vi "_DeviceCommandsInfo.vi"(0 "device name":string) -> (1 "error_stack":string[](array[string]), 2 "commands_info":T1(array[cluster]), 3 "success":bool=TRUE)   [LabVIEW 2014, in "tango.lvlib"]
uses:
  tango.lvlib
  tango_binding.so
panel:
  out "error_stack":string[](array[string])
  out "success":bool
  # "CommandInfo.level\n-----------------------\n\tOPERATOR = 0\n EXPERT = 1"
  # "CommandInfo.in-out-type\n-----------------------\n\tDEV_VOID = 0\n\tDEV_BOOLEAN = 1\n\tDEV_SHORT = 2\n\tDEV_LONG = 3\n\tDEV_FLOAT = 4\n\tDEV_DOUBLE = 5\n\tDEV_USHORT = 6\n\tDEV_ULONG = 7\n\tDEV_STRING = 8\n\tDEVVAR_CHARARRAY = 9\n\tDEVVAR_SHORTARRAY = 10\n\tDEVVAR_LONGARRAY = 11\n\tDEVVAR_FLOATARRAY = 12\n\tDEVVAR_DOUBLEARRAY = 13\n\tDEVVAR_USHORTARRAY = 14\n\tDEVVAR_ULONGARRAY = 15\n\tDEVVAR_STRINGARRAY = 16\n\tDEVVAR_LONGSTRINGARRAY = 17\n\tDEVVAR_DOUBLESTRINGARRAY = 18\n\tDEV_STATE = 19\n\tCONST_DEV_STRING = 20\n\tDEVVAR_BOOLEANARRAY = 21\n\tDEV_UCHAR = 22\n\tDEV_LONG64 = 23\n\tDEV_ULONG64 = 24\n\tDEVVAR_LONG64ARRAY = 25\n\tDEVVAR_ULONG64ARRAY = 26\n\tDEV_INT = 26\n\tDEV_ENCODED = 28"
  # "This Vi is deprecated and only maintained for backward compatibility. Please use  _TangoDeviceCommandsInfo instead."
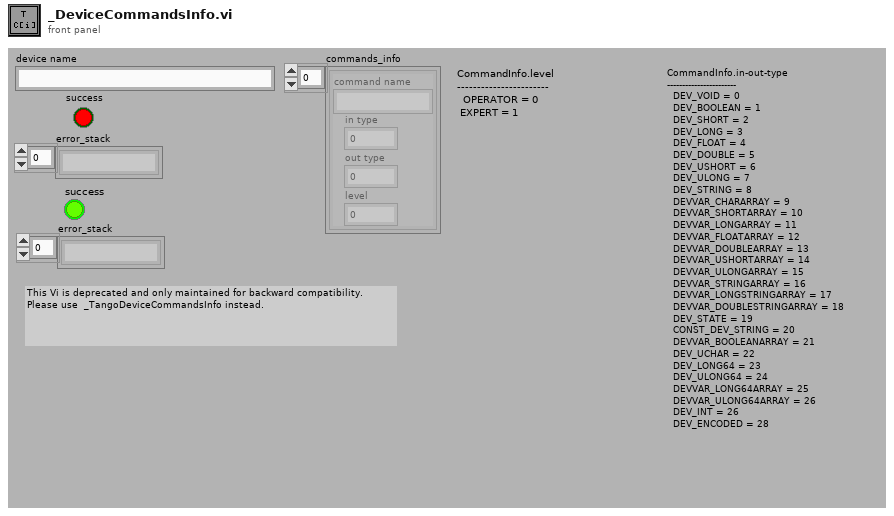
[diagram p1: front panel]
types:
  T1 = cluster{"command name":string, "in type":i16, "out type":i16, "level":i16}[]
  T2 = cluster{"command name":string, "in type":i16, "out type":i16, "level":i16}
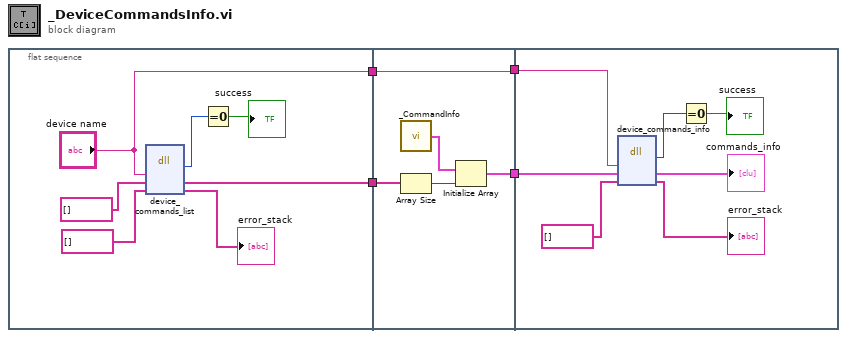
[diagram p0: block diagram]
diagram:
  n1 = flat-sequence {
    tunnel: [w7] -> w4
    tunnel: ["device name"] -> w3
    tunnel: w4 -> [w16]
    tunnel: [w13] -> w2
    tunnel: [w12] -> w1
    tunnel: w3 -> [w12]
    tunnel: w2 -> [w20]
    tunnel: w1 -> [w19]
    frame #0 {
      n2 = dll-call lib="tango_binding.*" fn="device_commands_list"("dev_name"="device name", "attributes_list"=string[] [] ("Error Stack"), "error_stack"=string[] [] ("Error Stack")) -> ("return type"=w9:i32, "attributes_list"=w7:string[], "error_stack"=→"error_stack":string[])  [unwired: 4 in, 2 out]
      n3 = Equal To 0?(x=w9) -> (x = 0?=→"success":bool)
    }
    frame #1 {
      n4 = call "_CommandInfo.vi"() -> ("command info"=w14:T2)
      n5 = Array Size(array=w16) -> (size(s)=w15:i32)
      n6 = Initialize Array(w14, w15) -> (w13:T1)
    }
    frame #2 {
      n7 = dll-call lib="tango_binding.*" fn="device_commands_info"("dev_name"=w19, "commands_info"=w20, "error_stack"=string[] [] ("Error Stack")) -> ("return type"=w21:i32, "commands_info"=→"commands_info":T1, "error_stack"=→"error_stack":string[])  [unwired: 4 in, 2 out]
      n8 = Equal To 0?(x=w21) -> (x = 0?=→"success":bool)
    }
  }
